vi "simulaFrec.vi"(8 "error in (no error)":errorcluster, 10 "frec in":dbl=0.75 format="%#_13g") -> (0 "error out":errorcluster, 2 "frec out":dbl)   [LabVIEW 2019, in "CNT90_GPIB.lvlib"]
uses:
  CNT90_GPIB.lvlib
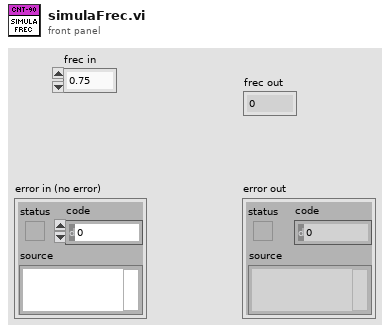
[diagram p1: front panel]
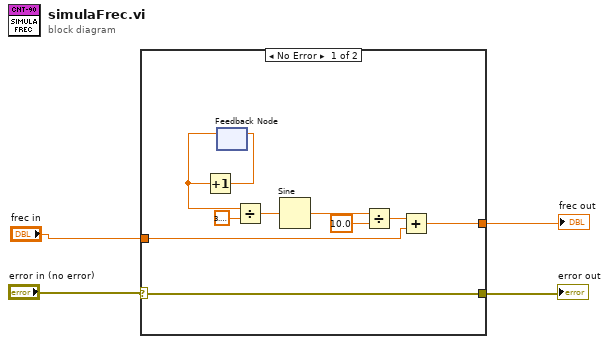
[diagram p0: block diagram]
diagram:
  n1 = case shown="No Error" "error in (no error)" {
    selector: "error in (no error)" -> [w7 w15]
    tunnel: [w7 w15] -> w3
    tunnel: "frec in" -> [w6 _]
    tunnel: [w5 _] -> w1
    frame No Error {
      n2 = feedback #1() -> (w10:dbl)  [unwired: 1 in]
      n3 = Increment(x=w10) -> (x+1=w14:dbl)
      n4 = feedback-in #1(w14) -> ()
      n5 = Divide(x=w10, y=3.141592653589793) -> (x/y=w13:dbl)
      n6 = Sine(x=w13) -> (sin(x)=w11:dbl)
      n7 = Divide(x=w11, y=10.0) -> (x/y=w9:dbl)
      n8 = Add(x=w9, y=w6) -> (x+y=w5:dbl)
    }
    frame Error {
    }
  }
  "error out" <- w3
  "frec out" <- w1
